vi "pop.vi"(2 "Before":dbl[](array[numeric])) -> (5 "Popped":dbl, 6 "After":dbl[](array[numeric]))   [LabVIEW 2009]
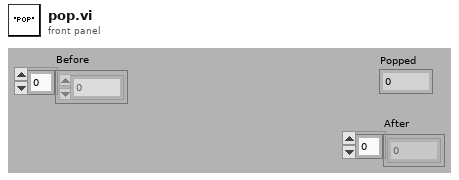
[diagram p1: front panel]
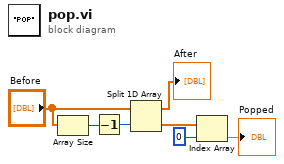
[diagram p0: block diagram]
diagram:
  n1 = Array Size(array="Before") -> (size(s)=w5:i32)
  n2 = Decrement(x=w5) -> (x-1=w4:i32)
  n3 = Split 1D Array(array="Before", index=w4) -> (first subarray=→"After":dbl[], second subarray=w3:dbl[])
  n4 = Index Array(array=w3, index=0) -> (element=→"Popped":dbl)
